vi "Command.vi"() -> ()   [LabVIEW 2017]
panel:
  out "Y-Feed":u32(slide) scale=0.0..10.0
  out "X-Feed":u32(slide)
  in  "Reset_Button":bool
  in  "Emergency":bool
  in  "Select_Mode":bool
  in  "Start_button":bool
  in  "Select_Model":enum32{"Manaul", "Automatic"}(tab)
  in  "Ref_Position_Y":i32[](array[numeric])=[28087, 16118, 3898, 0]
  in  "Ref_Position_X":i32[](array[numeric])=[20717, 17415, 14173, 11001, 7616, 0]
  # "Reset"
  # "Emergency"
  # "Manual"
  # "Auto"
  # "Start"
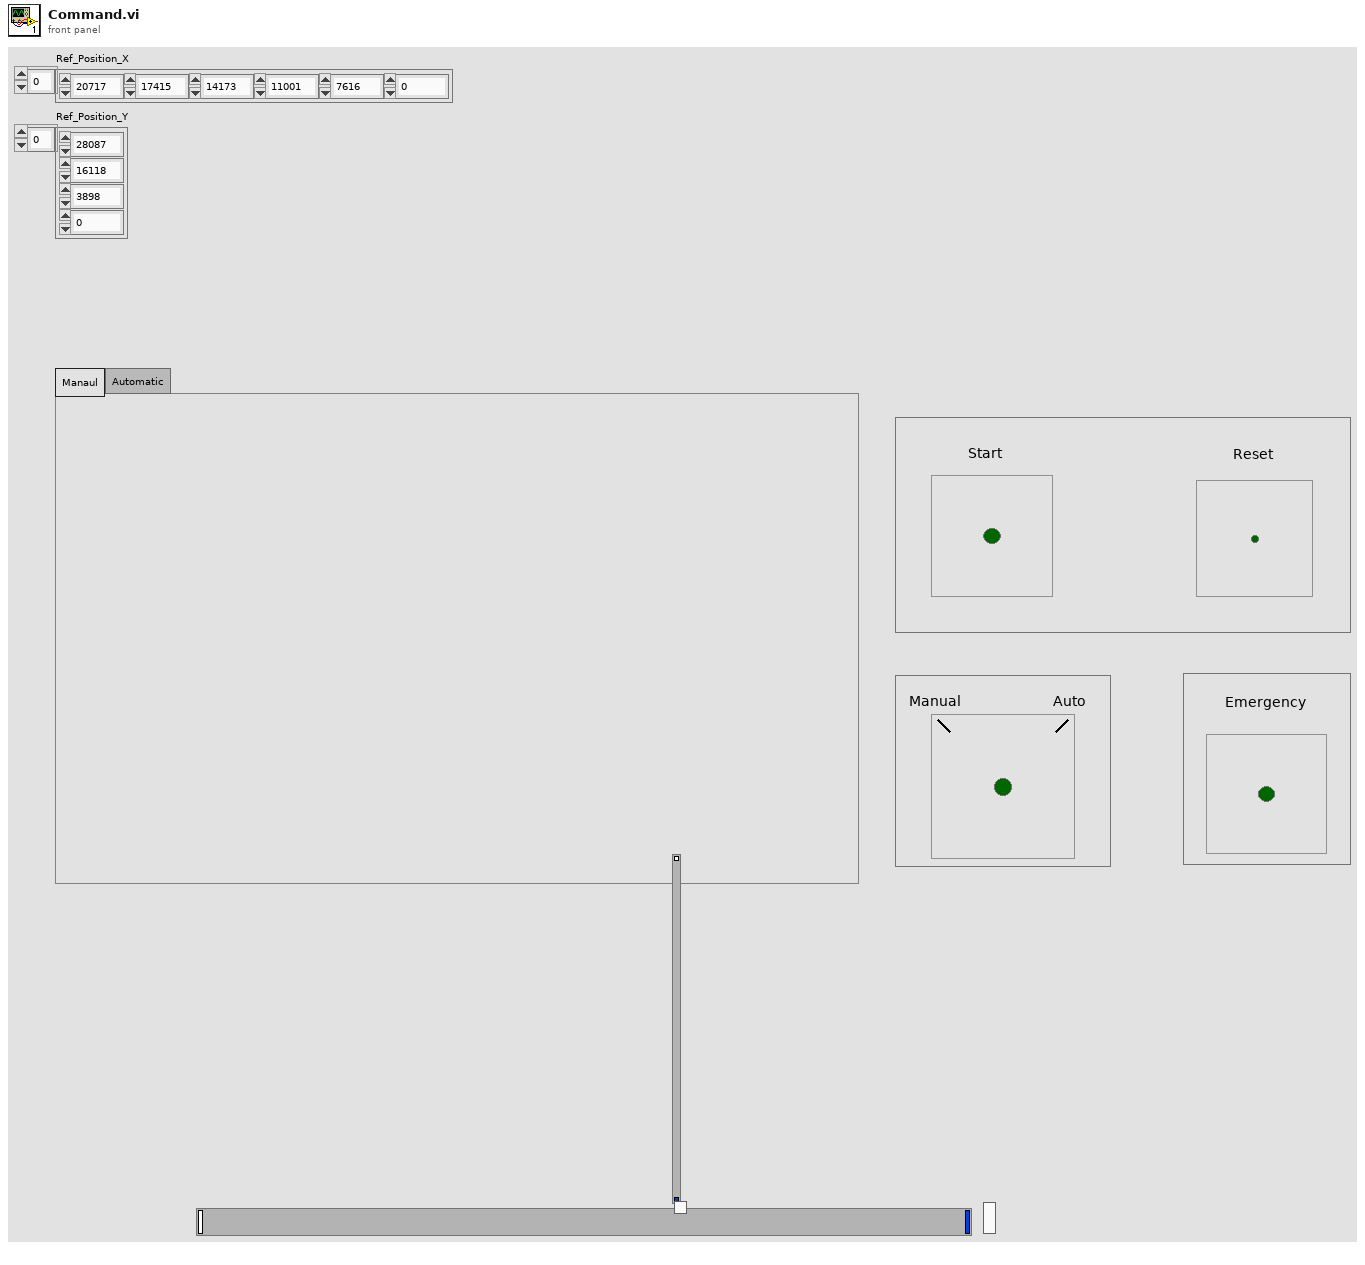
[diagram p1: front panel]
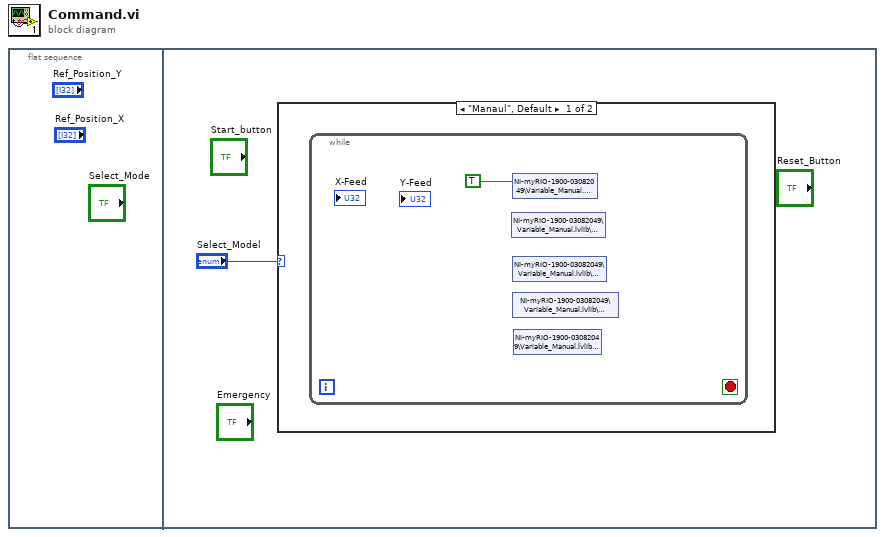
[diagram p0: block diagram]
diagram:
  n1 = flat-sequence {
    frame #0 {
    }
    frame #1 {
      n2 = case shown="\"Manaul\", Default" "Select_Model" {
        frame "Manaul", Default {
          n3 = while {
            stop <- _ stop-if-true
            n4 = shared-variable "NI-myRIO-1900-03082049\\Variable_Manual.lvlib\\X-Axis_M"() -> ()  [unwired: 2 in, 1 out]
            n5 = shared-variable "NI-myRIO-1900-03082049\\Variable_Manual.lvlib\\Start_M"(TRUE ("Start_M")) -> ()  [unwired: 1 in, 1 out]
            n6 = shared-variable "NI-myRIO-1900-03082049\\Variable_Manual.lvlib\\Y-Axis_M"() -> ()  [unwired: 2 in, 1 out]
            n7 = shared-variable "NI-myRIO-1900-03082049\\Variable_Manual.lvlib\\Retrieval_M"() -> ()  [unwired: 2 in, 1 out]
            n8 = shared-variable "NI-myRIO-1900-03082049\\Variable_Manual.lvlib\\Store_M"() -> ()  [unwired: 2 in, 1 out]
          }
        }
        frame "Automatic" {
        }
      }
    }
  }
